vi "Open.vi"(8 "error in (no error)":errorcluster, 10 "Create if not exists? (T)":bool=TRUE, 11 "Path":path) -> (0 "error out":errorcluster, 1 "File Exists?":bool, 2 "File Created?":bool, 3 "Config":T1)   [LabVIEW 2022 SP3, in "LabVIEW-Config.lvlib"]
uses:
  LabVIEW-Config.lvlib
  Config.ctl
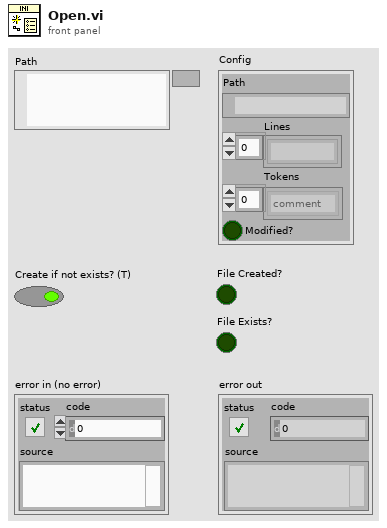
[diagram p1: front panel]
types:
  T1 = typedef "LabVIEW-Config.lvlib/Config.ctl" = cluster{"Path":path, "Lines":string[], "Tokens":enum8{"comment", "section", "key"}[], "Modified?":bool}
  T2 = enum16{"open", "replace", "create", "open or create", "replace or create", "replace or create with confirmation"}
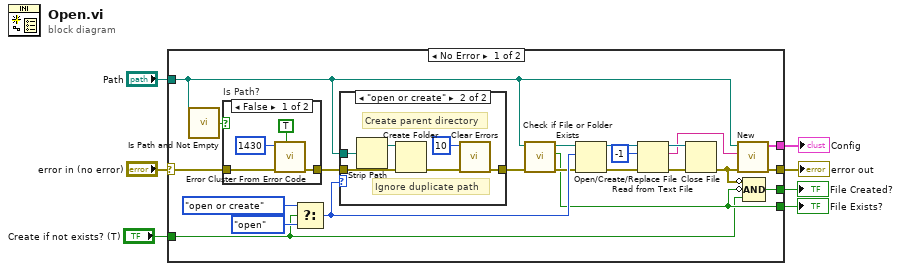
[diagram p0: block diagram]
diagram:
  n1 = case shown="No Error" "error in (no error)" {
    selector: "error in (no error)" -> [w24 w42]
    tunnel: [w10 _] -> w7
    tunnel: [w13 w42] -> w5
    tunnel: "Create if not exists? (T)" -> [w8 _]
    tunnel: "Path" -> [w11 _]
    tunnel: [w15 _] -> w2
    tunnel: [w14 _] -> w1
    frame No Error {
      n2 = call <vilib>:"Is Path and Not Empty.vi"("path"=w11) -> ("Is Path and Not Empty?"=w18:bool)  [unwired: 4 in]
      n3 = case "Is Path?" shown="False" w18 {
        tunnel: w24 -> [w33 w34]
        tunnel: [w31 w34] -> w21
        frame False {
          n4 = call <vilib>:"Error Cluster From Error Code.vi"("show call chain? (False)"=TRUE, "error in (no error)"=w33, "error code (0)"=1430) -> ("error out"=w31:errorcluster)  [unwired: 6 in]
        }
        frame True {
        }
      }
      n5 = Select(t=T2."open or create" ("operation (0:open)"), s=w8, f=T2."open" ("operation (0:open)")) -> (s? t:f=w19:T2)
      n6 = case shown="\"open or create\"" w19 {
        tunnel: w21 -> [w35 w41]
        tunnel: [w35 w36] -> w20
        tunnel: w11 -> [_ w40]
        frame Default {
        }
        frame "open or create" {
          # "Create parent directory"
          # "Ignore duplicate path"
          n7 = Strip Path(path=w40) -> (stripped path=w39:path)  [unwired: 1 out]
          n8 = Create Folder(path (use dialog)=w39, error in=w41) -> (error out=w37:errorcluster)  [unwired: 1 in, 2 out]
          n9 = call <vilib>:"Clear Errors.vi"("error in (no error)"=w37, "specific error code to clear (0: all)"=10 ("Not Found")) -> ("error out"=w36:errorcluster)  [unwired: 4 in, 1 out]
        }
      }
      n10 = call <vilib>:"Check if File or Folder Exists.vi"("error in (no error)"=w20, "path"=w11) -> ("error out"=w17:errorcluster, "file or folder exists?"=w15:bool, "dup path"=w16:path)  [unwired: 7 in]
      n11 = Open/Create/Replace File(file path (use dialog)=w16, error in=w17, operation (0:open)=w19) -> (refnum out=w26:refnum<file>, error out=w27:errorcluster)  [unwired: 3 in, 1 out]
      n12 = Read from Text File(file (use dialog)=w26, count=-1, error in=w27) -> (refnum out=w28:refnum<file>, text=w12:string, error out=w29:errorcluster)  [unwired: 1 in, 1 out]
      n13 = Close File(refnum=w28, error in=w29) -> (error out=w9:errorcluster)  [unwired: 1 out]
      n14 = call "New.vi"("error in (no error)"=w9, "Text"=w12, "Path (\"\")"=w11) -> ("error out"=w13:errorcluster, "Config"=w10:T1)  [unwired: 7 in]
      n15 = Compound Arithmetic op=AND(invert w9, invert w15, w8) -> (w14:bool)
    }
    frame Error {
    }
  }
  "error out" <- w5
  "Config" <- w7
  "File Exists?" <- w2
  "File Created?" <- w1
